vi "Find contact point.vi"(0 "reference in":refnum<class "Force Curve_tdms.lvclass">, 5 "error in (no error)":errorcluster, 7 "Signal in":T1=enum."SensorIn") -> (14 "reference out":refnum<class "Force Curve_tdms.lvclass">, 16 "contact index":i32, 19 "error out":errorcluster)   [LabVIEW 2019, in "Force Curve_tdms.lvclass"]
uses:
  Force Curve_tdms.lvclass
  Signal In.ctl
panel:
  out "Fcurve Metadata.Zpos contact":dbl
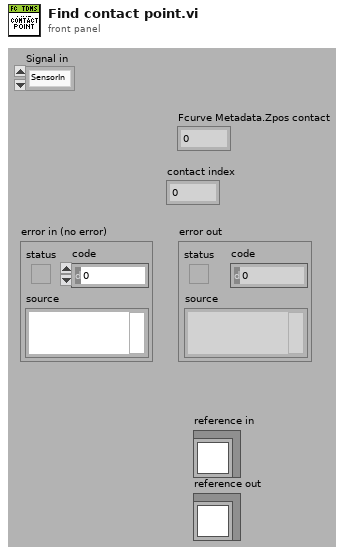
[diagram p1: front panel]
types:
  T1 = typedef "Force Curve_tdms.lvclass/Signal In.ctl" = enum16{"Deflection", "SensorIn", "MockOut", "ZstageOut"}
  T2 = typedef "Force Curve_tdms.lvclass/ObjectAttributes.ctl" = cluster{"MyAttribute":dbl, "Processed data":waveform(dbl)[], "Fcurve Raw Metadata":T3, "Fcurve Metadata":T4, "Fcurve index":T5, "Tau Delay (ms)":dbl, "Contact Spread of dev":dbl, "Fcurve":T6}
  T3 = typedef "TDMS_DataHandler.lvclass/Fcurve Meta data.ctl" = cluster{"property names":string[], "property values":variant[]}
  T4 = typedef "Force Curve_tdms.lvclass/Fcurve Meta data analysis.ctl" = cluster{"dt (us)":dbl, "Dec Factor":dbl, "Z piezo Sensitivity (nm/V)":dbl, "K (N/m)":dbl, "Sp (V)":dbl, "Contact (ms)":dbl, "Zpos contact":dbl, "Vel_app (nm/s)":dbl, "Vel_ret (nm/s)":dbl, "deltaV (nm)":dbl, "Def_V0 (v)":dbl, "Decimating Factor":dbl}
  T5 = typedef "Force Curve_tdms.lvclass/Fcurve Index .ctl" = cluster{"Setpoint index":i32, "Max force index":i32, "Contact point index":i32, "Appoach indices":cluster{"Start":i32, "End":i32}, "Contact indices":cluster{"Start":i32, "End":i32}, "Retract indices":cluster{"Start":i32, "End":i32}}
  T6 = typedef "Force Curve_tdms.lvclass/Force Curve data.ctl" = cluster{"Approach":cluster{"X":dbl[], "Y":dbl[]}, "Contact":cluster{"X":dbl[], "Y":dbl[]}, "Retract":cluster{"X":dbl[], "Y":dbl[]}}
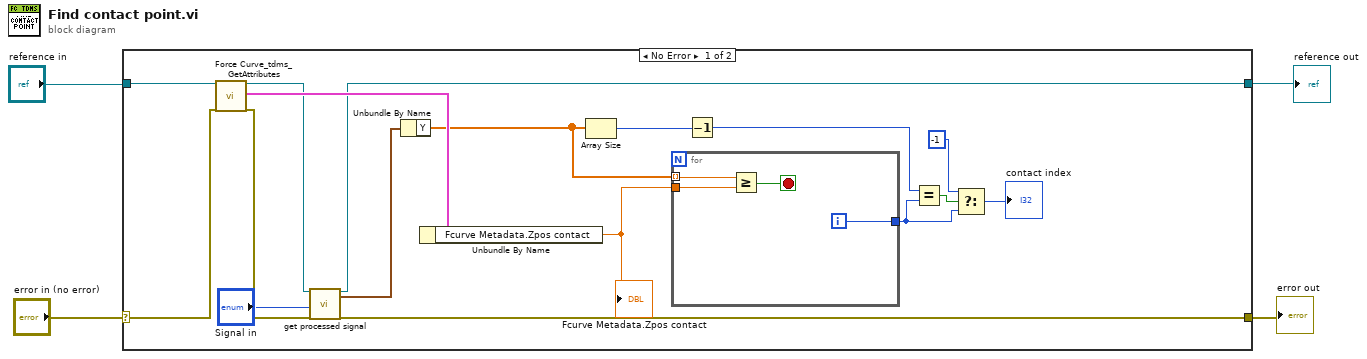
[diagram p0: block diagram]
diagram:
  n1 = case shown="No Error" "error in (no error)" {
    selector: "error in (no error)" -> [w15 w27]
    tunnel: [w10 w27] -> w3
    tunnel: "reference in" -> [w14 w26]
    tunnel: [w5 w26] -> w1
    frame No Error {
      n2 = call "Force Curve_tdms_GetAttributes.vi"("reference in"=w14, "error in (no error)"=w15) -> ("reference out"=w6:refnum<class "Force Curve_tdms.lvclass">, "attributes"=w13:T2, "error out"=w11:errorcluster)  [unwired: 14 in, 1 out]
      n3 = call "get processed signal.vi"("reference in"=w6, "error in (no error)"=w11, "Signal in"="Signal in") -> ("reference out"=w5:refnum<class "Force Curve_tdms.lvclass">, "Wfm out"=w7:waveform(dbl), "error out"=w10:errorcluster)  [unwired: 14 in]
      n4 = Unbundle By Name(w7) -> ("Y"=w9:dbl[])
      n5 = Unbundle By Name(w13) -> ("Fcurve Metadata.Zpos contact"=w12:dbl)
      "Fcurve Metadata.Zpos contact" <- w12
      n6 = Array Size(array=w9) -> (size(s)=w21:i32)
      n7 = for {
        tunnel: w9 -> [w25] mode=indexing
        tunnel: w12 -> [w24]
        tunnel: [w22] -> w18
        i -> [w22]
        stop <- w23 stop-if-true
        n8 = Greater Or Equal?(x=w25, y=w24) -> (x >= y?=w23:bool)
      }
      n9 = Decrement(x=w21) -> (x-1=w20:i32)
      n10 = Equal?(x=w20, y=w18) -> (x = y?=w19:bool)
      n11 = Select(t=-1, s=w19, f=w18) -> (s? t:f=→"contact index":i32)
    }
    frame Error {
    }
  }
  "error out" <- w3
  "reference out" <- w1
